vi "Create Execution.vi"(7 "Hierarchy":string, 8 "error in (no error)":errorcluster, 11 "Reg Notifier":refnum<notifier>) -> (0 "error out":errorcluster, 3 "Reg Event":refnum<user-event>)   [LabVIEW 2020, in "FlexBlocks.lvlib"]
uses:
  FlexBlocks.lvlib
  Execution Manager Async.vi
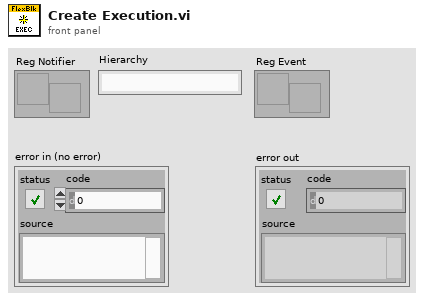
[diagram p1: front panel]
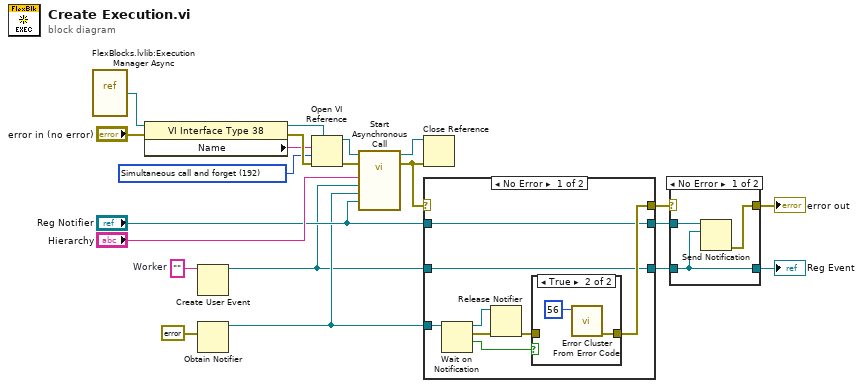
[diagram p0: block diagram]
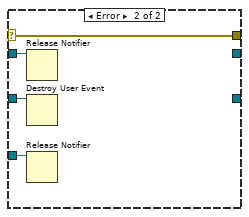
[diagram p3: hidden frame]
diagram:
  w2 = ""  # Worker
  w16 = 192 items=["Record modifications"=1, "Open templates for editing"=2, "Prompt user to save"=4, "Prepare for reentrant run"=8, "Prompt to find missing subVIs"=16, "Hide loading dialog box"=32, "Enable simultaneous calls"=64, "Prepare to call and forget"=128, "Simultaneous call and forget"=192, "Prepare to call and collect"=256, "Simultaneous call and collect"=320]
  n1 = vi-ref "FlexBlocks.lvlib:Execution Manager Async.vi"() -> (w14:refnum<vi>)
  n2 = property class="VI Interface Type 38"(reference=w14, error in="error in (no error)") -> (reference out=w17:refnum<vi>, error out=w21:errorcluster, "Name"=w15:string)
  n3 = Create User Event(user event datatype=w2) -> (user event=w1:refnum<user-event>)  [unwired: 1 in, 1 out]
  n4 = Obtain Notifier(notification data type=errorcluster {"status"=FALSE, "code"=0, "source"=""} ("error constant")) -> (notifier out=w9:refnum<notifier>)  [unwired: 3 in, 2 out]
  n5 = Open VI Reference(type specifier VI Refnum (for type only)=w17, vi path=w15, options=w16, error in (no error)=w21) -> (vi reference=w19:refnum<vi>, error out=w18:errorcluster)  [unwired: 2 in]
  n6 = call-by-ref "Start Asynchronous Call"(reference=w19, error in=w18, "Reg Notifier"="Reg Notifier", "Ready Handshake"=w9, "Reg Event"=w1, "Hierarchy"="Hierarchy") -> (reference out=w20:refnum<vi>, error out=w11:errorcluster)  [unwired: 8 in]
  n7 = Close Reference(reference=w20, error in (no error)=w11) -> ()  [unwired: 1 out]
  n8 = case shown="No Error" w11 {
    selector: w11 -> [_ w36]
    tunnel: "Reg Notifier" -> [w22 w33]
    tunnel: w9 -> [w29 w34]
    tunnel: w1 -> [w23 w35]
    tunnel: [w24 w36] -> w8
    tunnel: [w23 _] -> w7
    tunnel: [w22 _] -> w6
    frame No Error {
      n9 = Wait on Notification(notifier=w29) -> (notifier out=w27:refnum<notifier>, notification=w26:errorcluster, timed out?=w28:bool)  [unwired: 3 in, 1 out]
      n10 = Release Notifier(notifier=w27, error in (no error)=w26) -> (error out=w25:errorcluster)  [unwired: 1 in, 2 out]
      n11 = case shown="True" w28 {
        tunnel: w25 -> [w30 _]
        tunnel: [w30 w31] -> w24
        frame False {
        }
        frame True {
          n12 = call <vilib>:"Error Cluster From Error Code.vi"("error code (0)"=56) -> ("error out"=w31:errorcluster)  [unwired: 8 in]
        }
      }
    }
    frame Error {
      n13 = Release Notifier(notifier=w33) -> ()  [unwired: 2 in, 3 out]
      n14 = Destroy User Event(user event=w35) -> ()  [unwired: 1 in, 1 out]
      n15 = Release Notifier(notifier=w34) -> ()  [unwired: 2 in, 3 out]
    }
  }
  n16 = case shown="No Error" w8 {
    selector: w8 -> [_ w40]
    tunnel: w6 -> [w39 _]
    tunnel: w7 -> [w38 _]
    tunnel: [w37 w40] -> w5
    tunnel: [w38 _] -> w4
    frame No Error {
      n17 = Send Notification(notification=w38, notifier=w39) -> (error out=w37:errorcluster)  [unwired: 1 in, 1 out]
    }
    frame Error {
    }
  }
  "error out" <- w5
  "Reg Event" <- w4
